vi "list_all_switch_chan_states_names.vi"(8 "error in (no error)":errorcluster) -> (0 "error out":errorcluster, 2 "switch info":T1)   [LabVIEW 2015]
doc: "goes through all PrepLineObjects and lists all switch channels and the Instrument that belongs to them as well as the state of each switch"
uses:
  global variables.vi
  PrepLineObject.lvclass
  StatusLog/StatusLog.lvclass
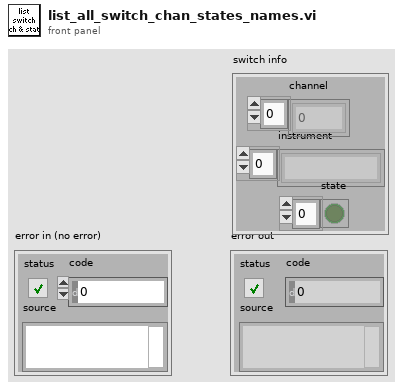
[diagram p1: front panel]
types:
  T1 = cluster{"channel":u16[], "instrument":string[], "state":bool[]}
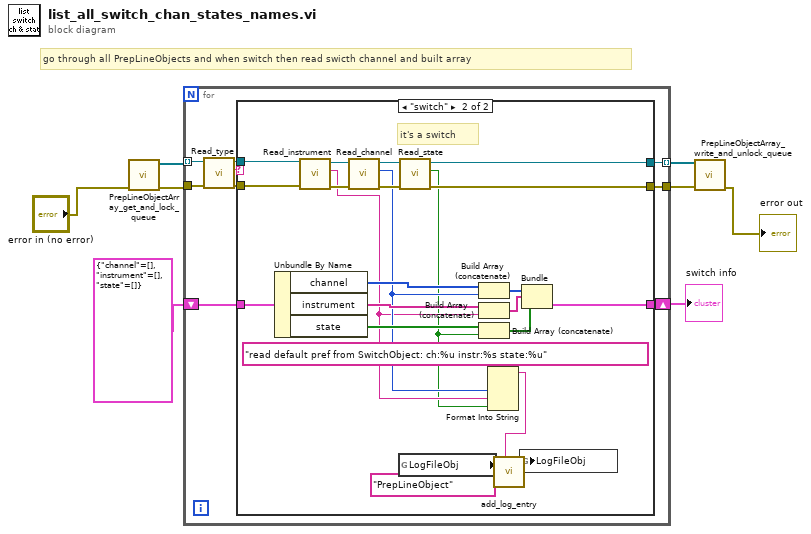
[diagram p0: block diagram]
diagram:
  # "go through all PrepLineObjects and when switch then read swicth channel and built array"
  n1 = call "PrepLineObjectArray_get_and_lock_queue.vi"("error in (no error)"="error in (no error)") -> ("error out"=w5:errorcluster, "PrepLineObjects"=w4:refnum<class "PrepLineObject.lvclass">[])  [unwired: 9 in]
  n2 = for {
    tunnel: w4 -> [w17] mode=indexing
    shift-right: [w12] -> w7
    shift-left: T1 {"channel"=[], "instrument"=[], "state"=[]} -> [w16]
    tunnel: w5 -> [w11]
    tunnel: [w10] -> w3
    tunnel: [w9] -> w2 mode=indexing
    n3 = call-dynamic "Read_type.vi"("error in (no error)"=w11, "PrepLinePictureObjects in"=w17) -> ("error out"=w13:errorcluster, "String"=w15:string, "PrepLinePictureObjects out"=w14:refnum<class "PrepLineObject.lvclass">)  [unwired: 7 in]
    n4 = case shown="\"switch\"" w15 {
      tunnel: w16 -> [w20 w40]
      tunnel: w14 -> [w18 w44]
      tunnel: w13 -> [w19 w42]
      tunnel: [w20 w35] -> w12
      tunnel: [w19 w32] -> w10
      tunnel: [w18 w21] -> w9
      frame "False", Default {
      }
      frame "switch" {
        # "it's a switch"
        n5 = Unbundle By Name(w40) -> ("channel"=w39:u16[], "instrument"=w38:string[], "state"=w31:bool[])
        n6 = call-dynamic "Read_instrument.vi"("PrepLinePictureObjects in"=w44, "error in (no error)"=w42) -> ("PrepLinePictureObjects out"=w43:refnum<class "PrepLineObject.lvclass">, "instrument name"=w25:string, "error out"=w41:errorcluster)  [unwired: 6 in]
        n7 = call-dynamic "Read_channel.vi"("error in (no error)"=w41, "PrepLineObject in"=w43) -> ("error out"=w33:errorcluster, "channel"=w26:u16, "PrepLineObject out"=w34:refnum<class "PrepLineObject.lvclass">)  [unwired: 7 in]
        n8 = global read "global variables.vi" "LogFileObj"() -> (w29:refnum<class "StatusLog.lvclass">)
        n9 = call-dynamic "Read_state.vi"("error in (no error)"=w33, "PrepLineObject in"=w34) -> ("error out"=w32:errorcluster, "state"=w24:bool, "PrepLineObject out"=w21:refnum<class "PrepLineObject.lvclass">)  [unwired: 7 in]
        n10 = Build Array (concatenate)(w39, w26) -> (w37:u16[])
        n11 = Build Array (concatenate)(w38, w25) -> (w36:string[])
        n12 = Build Array (concatenate)(w31, w24) -> (w30:bool[])
        n13 = Format Into String(format string="read default pref from SwitchObject: ch:%u instr:%s state:%u", w26, w25, w24) -> (resulting string=w23:string)  [unwired: 2 in, 1 out]
        n14 = call-dynamic "add_log_entry.vi"("new entry"=w23, "log identifiers"="PrepLineObject", "StatusLog in"=w29) -> ("StatusLog out"=w28:refnum<class "StatusLog.lvclass">)  [unwired: 5 in, 1 out]
        n15 = global write "global variables.vi" "LogFileObj"(w28) -> ()
        n16 = Bundle(w37, w36, w30) -> (w35:cluster{u16[], string[], bool[]})  [unwired: 1 in]
      }
    }
  }
  "switch info" <- w7
  n17 = call "PrepLineObjectArray_write_and_unlock_queue.vi"("error in (no error)"=w3, "PrepLineObjArray"=w2) -> ("error out"=→"error out":errorcluster)  [unwired: 9 in]
